vi "fxpConfigureOverflowMode.vi"(8 "error in":errorcluster, 10 "fxpXctl refnums":T1, 11 "Display State In":T2) -> (0 "error out":errorcluster)   [LabVIEW 2020, in "FXP.xctl"]
uses:
  <vilib>/fxp/FXPxcontrol/FXP.xctl
  <vilib>/fxp/FXPxcontrol/fxpState.ctl
  <vilib>/fxp/LVFixedPointQuantizationPolicyTypeDef.ctl
  <vilib>/fxp/LVFixedPointOverflowPolicyTypeDef.ctl
  <vilib>/fxp/FXPxcontrol/fxpChangeEvent.ctl
  <vilib>/fxp/FXPxcontrol/fxpValueChangeControl.ctl
  <vilib>/fxp/FXPxcontrol/fxpMixedStateStatus.ctl
  <vilib>/fxp/FXPxcontrol/fxpFacadeCtlRefnums.ctl
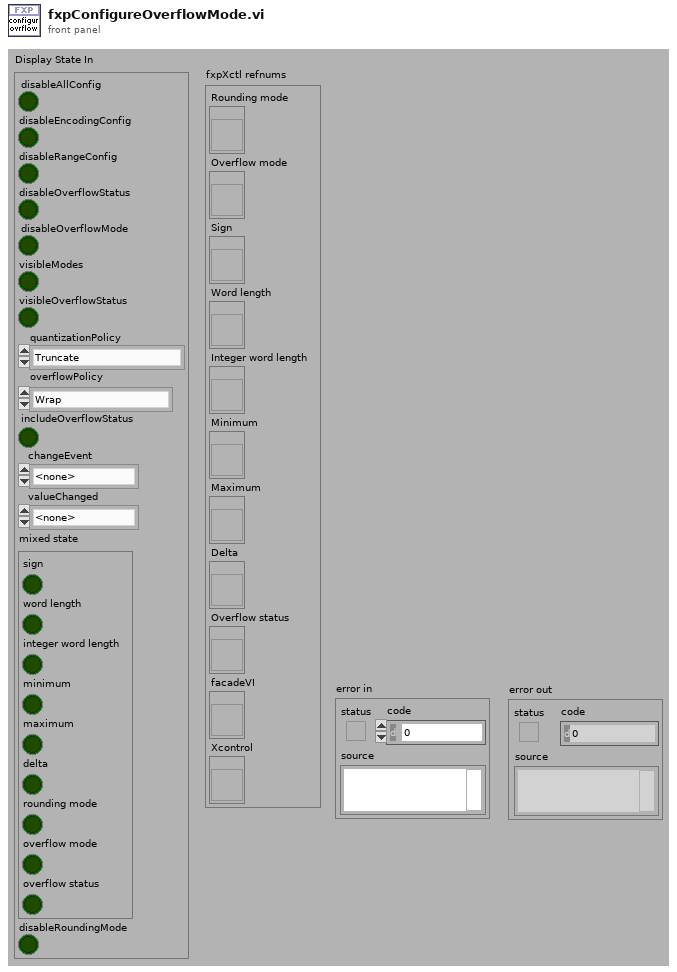
[diagram p1: front panel]
types:
  T1 = typedef "FXP.xctl/fxpFacadeCtlRefnums.ctl" = cluster{"Rounding mode":refnum<vi>, "Overflow mode":refnum<vi>, "Sign":refnum<vi>, "Word length":refnum<vi>, "Integer word length":refnum<vi>, "Minimum":refnum<vi>, "Maximum":refnum<vi>, "Delta":refnum<vi>, "Overflow status":refnum<vi>, "facadeVI":refnum<vi>, "Xcontrol":refnum<vi>}
  T2 = typedef "FXP.xctl/fxpState.ctl" = cluster{"disableAllConfig":bool, "disableEncodingConfig":bool, "disableRangeConfig":bool, "disableOverflowStatus":bool, "disableOverflowMode":bool, "visibleModes":bool, "visibleOverflowStatus":bool, "quantizationPolicy":T3, "overflowPolicy":T4, "includeOverflowStatus":bool, "changeEvent":T5, "valueChanged":T6, "mixed state":T7, "disableRoundingMode":bool}
  T3 = typedef "LVFixedPointQuantizationPolicyTypeDef.ctl" = enum32{"Truncate", "Round-Half-Up (Asymmetric)", "Round-Half-Even"}
  T4 = typedef "LVFixedPointOverflowPolicyTypeDef.ctl" = enum32{"Wrap", "Saturate"}
  T5 = typedef "FXP.xctl/fxpChangeEvent.ctl" = enum16{"<none>", "initialize", "modesVisible", "overflowModeEnabled", "overflowStatusVisible", "configEnabled", "modeRounding", "modeOverflow", "statusOverflow", "mixedState", "roundingModeEnabled"}
  T6 = typedef "FXP.xctl/fxpValueChangeControl.ctl" = enum16{"<none>", "sign", "word length", "integer word length", "minimum", "maximum", "delta", "rounding mode", "overflow mode", "overflow status"}
  T7 = typedef "FXP.xctl/fxpMixedStateStatus.ctl" = cluster{"sign":bool, "word length":bool, "integer word length":bool, "minimum":bool, "maximum":bool, "delta":bool, "rounding mode":bool, "overflow mode":bool, "overflow status":bool}
  T8 = enum8{"Enabled", "Disabled", "Disabled and Grayed Out"}
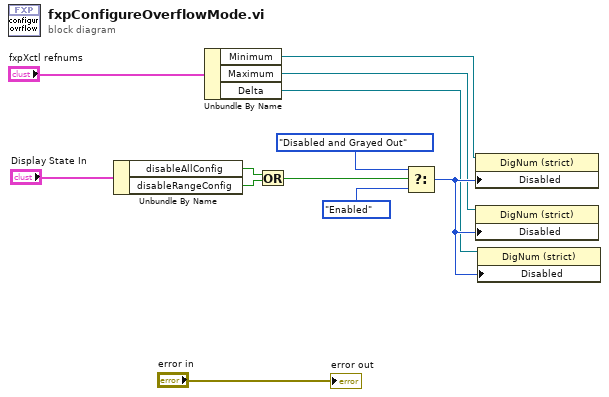
[diagram p0: block diagram]
diagram:
  n1 = Unbundle By Name("Display State In") -> ("disableAllConfig"=w5:bool, "disableRangeConfig"=w1:bool)
  n2 = Unbundle By Name("fxpXctl refnums") -> ("Minimum"=w9:refnum<vi>, "Maximum"=w8:refnum<vi>, "Delta"=w7:refnum<vi>)
  n3 = Or(x=w5, y=w1) -> (x .or. y?=w4:bool)
  n4 = Select(t=T8."Disabled and Grayed Out" ("Disabled"), s=w4, f=T8."Enabled" ("Disabled")) -> (s? t:f=w12:T8)
  n5 = property on="Property Node" class="DigNum (strict)"(reference=w9, "Disabled"=w12) -> ()  [unwired: 1 in, 2 out]
  n6 = property on="Property Node" class="DigNum (strict)"(reference=w8, "Disabled"=w12) -> ()  [unwired: 1 in, 2 out]
  n7 = property on="Property Node" class="DigNum (strict)"(reference=w7, "Disabled"=w12) -> ()  [unwired: 1 in, 2 out]
  "error out" <- "error in"
